vi "Write Start Homing.vi"(8 "error in (no error)":errorcluster, 10 "Start":bool, 11 "FHPP in":refnum<class "FHPP.lvclass">) -> (0 "error out":errorcluster, 3 "FHPP out":refnum<class "FHPP.lvclass">)   [LabVIEW 2022 SP3, in "FHPP.lvclass"]
uses:
  FHPP.lvclass
  FHPP.lvclass/FHPP.ctl
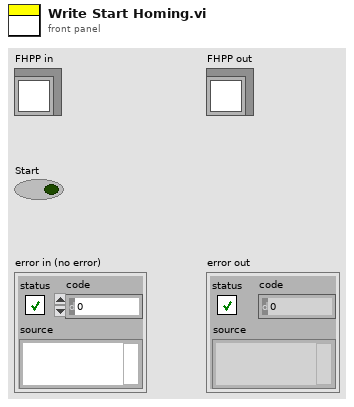
[diagram p1: front panel]
types:
  T1 = typedef "FHPP.lvclass/CPOS.ctl" = cluster{"Halt":bool, "Start":bool, "Start Homing":bool, "Jog Positive":bool, "Jog Negative":bool, "Teach Actual Value":bool, "Clear Remaining Pos":bool, "Reserved":bool}
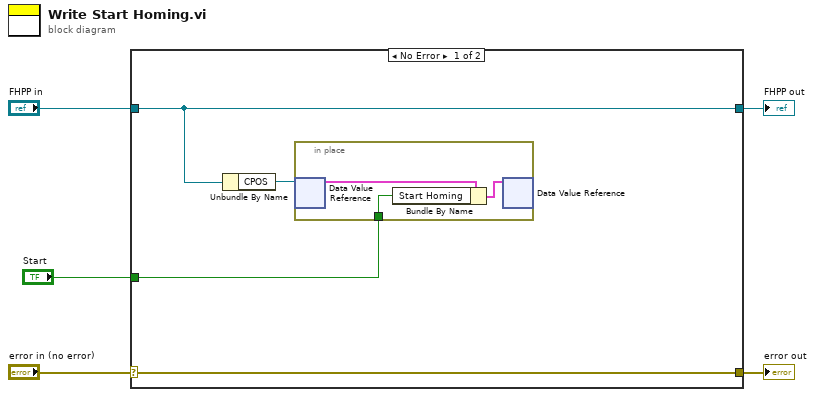
[diagram p0: block diagram]
diagram:
  n1 = case shown="No Error" "error in (no error)" {
    selector: "error in (no error)" -> [w9 w14]
    tunnel: [w9 w14] -> w4
    tunnel: [w8 w13] -> w2
    tunnel: "FHPP in" -> [w8 w13]
    tunnel: "Start" -> [w6 _]
    frame No Error {
      n2 = Unbundle By Name(w8) -> ("CPOS"=w7:refnum<data-value>)
      n3 = in-place {
        in-place-border: w6 -> [w10]
        n4 = in-place-dvr #1(w7) -> (w12:T1)  [unwired: 1 out]
        n5 = Bundle By Name(cluster=w12, "Start Homing"=w10) -> (w11:T1)
        n6 = in-place-dvr #1(w11) -> ()  [unwired: 2 out]
      }
    }
    frame Error {
    }
  }
  "error out" <- w4
  "FHPP out" <- w2
